vi "ConvertTextBasedCodeToLabVIEW_CreateOverviewHtmlFile.vi"(5 "InterfacesThatWillUseInheritance":string[](array[string]), 7 "MissingClasses":string[](array[string]), 8 "error in (no error)":errorcluster, 10 "Classes":T1[](array[typedef])=[{"ClassName"="Global", "AccessScope"=enum."public", "Modifiers"=[enum."static", enum."const"], "ClassDocumentation"="", "Methods"=[{"ReturnType"={"Name"="", "DataType"=enum."UINT8", "ArrayDim"=0, "CtrlPath"=path "", "DataTypeString"="", "AccessScope"=enum."public", "InitialData"=variant}, "MethodName"="", "AccessScope"=enum."public", "Modifiers"=[], "MethodDocumentation"="", "MethodContent"="", "MethodArguments"=[], "GetProperty"={"Active"=FALSE, "AccessScope"=enum."public", "Code"=""}, "SetProperty"={"Active"=FALSE, "AccessScope"=enum."public", "Code"=""}}], "ParentClasses"=[{"ClassName"="HttpApplication", "ClassType"=enum."Undefined"}], "ClassType"=enum."Class", "Owner"="", "OwnerType"=enum."NoOwner", "Generics"=["X", "Y"], "Attributes"=[{"Name"="Name", "DataType"=enum."STRING", "ArrayDim"=0, "CtrlPath"=path "", "DataTypeString"="", "AccessScope"=enum."public", "InitialData"=variant}, {"Name"="Points", "DataType"=enum."Other", "ArrayDim"=1, "CtrlPath"=path "", "DataTypeString"="", "AccessScope"=enum."protected", "InitialData"=variant}], "Enums"=[{"Name"="Alignment", "AccessScope"=enum."public", "Modifiers"=[], "Items"=["Top", "Left"], "Documentation"="This is doc"}], "Structs"=[{"Name"="MyStruct", "AccessScope"=enum."public", "Modifiers"=[enum."static"], "Items"=[{"Name"="A", "DataType"=enum."UINT8", "ArrayDim"=0, "CtrlPath"=path "", "DataTypeString"="", "AccessScope"=enum."public", "InitialData"=variant}, {"Name"="B", "DataType"=enum."INT32", "ArrayDim"=2, "CtrlPath"=path "", "DataTypeString"="", "AccessScope"=enum."public", "InitialData"=variant}], "Documentation"="Doc of My Strcutc\nBlah Blah YUmmi"}]}, {"ClassName"="ApplicationUser", "AccessScope"=enum."public", "Modifiers"=[], "ClassDocumentation"="You can add User data for the user by adding more properties to your User class, please visit http://    public", "Methods"=[{"ReturnType"={"Name"="", "DataType"=enum."UINT8", "ArrayDim"=0, "CtrlPath"=path "", "DataTypeString"="", "AccessScope"=enum."public", "InitialData"=variant}, "MethodName"="", "AccessScope"=enum."public", "Modifiers"=[], "MethodDocumentation"="", "MethodContent"="", "MethodArguments"=[], "GetProperty"={"Active"=FALSE, "AccessScope"=enum."public", "Code"=""}, "SetProperty"={"Active"=FALSE, "AccessScope"=enum."public", "Code"=""}}, {"ReturnType"={"Name"="", "DataType"=enum."UINT8", "ArrayDim"=0, "CtrlPath"=path "", "DataTypeString"="", "AccessScope"=enum."public", "InitialData"=variant}, "MethodName"="", "AccessScope"=enum."public", "Modifiers"=[], "MethodDocumentation"="", "MethodContent"="", "MethodArguments"=[], "GetProperty"={"Active"=FALSE, "AccessScope"=enum."public", "Code"=""}, "SetProperty"={"Active"=FALSE, "AccessScope"=enum."public", "Code"=""}}], "ParentClasses"=[{"ClassName"="IdentityUser", "ClassType"=enum."Undefined"}], "ClassType"=enum."Class", "Owner"="", "OwnerType"=enum."NoOwner", "Generics"=[], "Attributes"=[], "Enums"=[], "Structs"=[]}, {"ClassName"="ApplicationDbContext", "AccessScope"=enum."public", "Modifiers"=[], "ClassDocumentation"="", "Methods"=[{"ReturnType"={"Name"="", "DataType"=enum."UINT8", "ArrayDim"=0, "CtrlPath"=path "", "DataTypeString"="", "AccessScope"=enum."public", "InitialData"=variant}, "MethodName"="", "AccessScope"=enum."public", "Modifiers"=[], "MethodDocumentation"="", "MethodContent"="", "MethodArguments"=[], "GetProperty"={"Active"=FALSE, "AccessScope"=enum."public", "Code"=""}, "SetProperty"={"Active"=FALSE, "AccessScope"=enum."public", "Code"=""}}, {"ReturnType"={"Name"="", "DataType"=enum."UINT8", "ArrayDim"=0, "CtrlPath"=path "", "DataTypeString"="", "AccessScope"=enum."public", "InitialData"=variant}, "MethodName"="", "AccessScope"=enum."public", "Modifiers"=[], "MethodDocumentation"="", "MethodContent"="", "MethodArguments"=[], "GetProperty"={"Active"=FALSE, "AccessScope"=enum."public", "Code"=""}, "SetProperty"={"Active"=FALSE, "AccessScope"=enum."public", "Code"=""}}], "ParentClasses"=[{"ClassName"="IdentityDbContext", "ClassType"=enum."Undefined"}], "ClassType"=enum."Class", "Owner"="", "OwnerType"=enum."NoOwner", "Generics"=["ApplicationUser"], "Attributes"=[], "Enums"=[], "Structs"=[]}, {"ClassName"="IdentityHelper", "AccessScope"=enum."public", "Modifiers"=[enum."static"], "ClassDocumentation"="", "Methods"=[{"ReturnType"={"Name"="", "DataType"=enum."UINT8", "ArrayDim"=0, "CtrlPath"=path "", "DataTypeString"="", "AccessScope"=enum."public", "InitialData"=variant}, "MethodName"="", "AccessScope"=enum."public", "Modifiers"=[], "MethodDocumentation"="", "MethodContent"="", "MethodArguments"=[], "GetProperty"={"Active"=FALSE, "AccessScope"=enum."public", "Code"=""}, "SetProperty"={"Active"=FALSE, "AccessScope"=enum."public", "Code"=""}}, {"ReturnType"={"Name"="", "DataType"=enum."UINT8", "ArrayDim"=0, "CtrlPath"=path "", "DataTypeString"="", "AccessScope"=enum."public", "InitialData"=variant}, "MethodName"="", "AccessScope"=enum."public", "Modifiers"=[], "MethodDocumentation"="", "MethodContent"="", "MethodArguments"=[], "GetProperty"={"Active"=FALSE, "AccessScope"=enum."public", "Code"=""}, "SetProperty"={"Active"=FALSE, "AccessScope"=enum."public", "Code"=""}}, {"ReturnType"={"Name"="", "DataType"=enum."UINT8", "ArrayDim"=0, "CtrlPath"=path "", "DataTypeString"="", "AccessScope"=enum."public", "InitialData"=variant}, "MethodName"="", "AccessScope"=enum."public", "Modifiers"=[], "MethodDocumentation"="", "MethodContent"="", "MethodArguments"=[], "GetProperty"={"Active"=FALSE, "AccessScope"=enum."public", "Code"=""}, "SetProperty"={"Active"=FALSE, "AccessScope"=enum."public", "Code"=""}}, {"ReturnType"={"Name"="", "DataType"=enum."UINT8", "ArrayDim"=0, "CtrlPath"=path "", "DataTypeString"="", "AccessScope"=enum."public", "InitialData"=variant}, "MethodName"="", "AccessScope"=enum."public", "Modifiers"=[], "MethodDocumentation"="", "MethodContent"="", "MethodArguments"=[], "GetProperty"={"Active"=FALSE, "AccessScope"=enum."public", "Code"=""}, "SetProperty"={"Active"=FALSE, "AccessScope"=enum."public", "Code"=""}}, {"ReturnType"={"Name"="", "DataType"=enum."UINT8", "ArrayDim"=0, "CtrlPath"=path "", "DataTypeString"="", "AccessScope"=enum."public", "InitialData"=variant}, "MethodName"="", "AccessScope"=enum."public", "Modifiers"=[], "MethodDocumentation"="", "MethodContent"="", "MethodArguments"=[], "GetProperty"={"Active"=FALSE, "AccessScope"=enum."public", "Code"=""}, "SetProperty"={"Active"=FALSE, "AccessScope"=enum."public", "Code"=""}}, {"ReturnType"={"Name"="", "DataType"=enum."UINT8", "ArrayDim"=0, "CtrlPath"=path "", "DataTypeString"="", "AccessScope"=enum."public", "InitialData"=variant}, "MethodName"="", "AccessScope"=enum."public", "Modifiers"=[], "MethodDocumentation"="", "MethodContent"="", "MethodArguments"=[], "GetProperty"={"Active"=FALSE, "AccessScope"=enum."public", "Code"=""}, "SetProperty"={"Active"=FALSE, "AccessScope"=enum."public", "Code"=""}}, {"ReturnType"={"Name"="", "DataType"=enum."UINT8", "ArrayDim"=0, "CtrlPath"=path "", "DataTypeString"="", "AccessScope"=enum."public", "InitialData"=variant}, "MethodName"="", "AccessScope"=enum."public", "Modifiers"=[], "MethodDocumentation"="", "MethodContent"="", "MethodArguments"=[], "GetProperty"={"Active"=FALSE, "AccessScope"=enum."public", "Code"=""}, "SetProperty"={"Active"=FALSE, "AccessScope"=enum."public", "Code"=""}}, {"ReturnType"={"Name"="", "DataType"=enum."UINT8", "ArrayDim"=0, "CtrlPath"=path "", "DataTypeString"="", "AccessScope"=enum."public", "InitialData"=variant}, "MethodName"="", "AccessScope"=enum."public", "Modifiers"=[], "MethodDocumentation"="", "MethodContent"="", "MethodArguments"=[], "GetProperty"={"Active"=FALSE, "AccessScope"=enum."public", "Code"=""}, "SetProperty"={"Active"=FALSE, "AccessScope"=enum."public", "Code"=""}}], "ParentClasses"=[], "ClassType"=enum."Class", "Owner"="", "OwnerType"=enum."NoOwner", "Generics"=[], "Attributes"=[{"Name"="XsrfKey", "DataType"=enum."STRING", "ArrayDim"=0, "CtrlPath"=path "", "DataTypeString"="string", "AccessScope"=enum."public", "InitialData"=variant(string "\"XsrfId\"")}, {"Name"="ProviderNameKey", "DataType"=enum."STRING", "ArrayDim"=0, "CtrlPath"=path "", "DataTypeString"="string", "AccessScope"=enum."public", "InitialData"=variant(string "\"providerName\"")}, {"Name"="CodeKey", "DataType"=enum."STRING", "ArrayDim"=0, "CtrlPath"=path "", "DataTypeString"="string", "AccessScope"=enum."public", "InitialData"=variant(string "\"code\"")}, {"Name"="UserIdKey", "DataType"=enum."STRING", "ArrayDim"=0, "CtrlPath"=path "", "DataTypeString"="string", "AccessScope"=enum."public", "InitialData"=variant(string "\"userId\"")}], "Enums"=[], "Structs"=[]}, {"ClassName"="Register", "AccessScope"=enum."public", "Modifiers"=[enum."partial"], "ClassDocumentation"="", "Methods"=[{"ReturnType"={"Name"="", "DataType"=enum."UINT8", "ArrayDim"=0, "CtrlPath"=path "", "DataTypeString"="", "AccessScope"=enum."public", "InitialData"=variant}, "MethodName"="", "AccessScope"=enum."public", "Modifiers"=[], "MethodDocumentation"="", "MethodContent"="", "MethodArguments"=[], "GetProperty"={"Active"=FALSE, "AccessScope"=enum."public", "Code"=""}, "SetProperty"={"Active"=FALSE, "AccessScope"=enum."public", "Code"=""}}, {"ReturnType"={"Name"="", "DataType"=enum."UINT8", "ArrayDim"=0, "CtrlPath"=path "", "DataTypeString"="", "AccessScope"=enum."public", "InitialData"=variant}, "MethodName"="", "AccessScope"=enum."public", "Modifiers"=[], "MethodDocumentation"="", "MethodContent"="", "MethodArguments"=[], "GetProperty"={"Active"=FALSE, "AccessScope"=enum."public", "Code"=""}, "SetProperty"={"Active"=FALSE, "AccessScope"=enum."public", "Code"=""}}], "ParentClasses"=[{"ClassName"="Page", "ClassType"=enum."Undefined"}], "ClassType"=enum."Class", "Owner"="", "OwnerType"=enum."NoOwner", "Generics"=[], "Attributes"=[], "Enums"=[], "Structs"=[]}, {"ClassName"="RoleActions", "AccessScope"=enum."internal", "Modifiers"=[], "ClassDocumentation"="", "Methods"=[{"ReturnType"={"Name"="", "DataType"=enum."UINT8", "ArrayDim"=0, "CtrlPath"=path "", "DataTypeString"="", "AccessScope"=enum."public", "InitialData"=variant}, "MethodName"="", "AccessScope"=enum."public", "Modifiers"=[], "MethodDocumentation"="", "MethodContent"="", "MethodArguments"=[], "GetProperty"={"Active"=FALSE, "AccessScope"=enum."public", "Code"=""}, "SetProperty"={"Active"=FALSE, "AccessScope"=enum."public", "Code"=""}}], "ParentClasses"=[], "ClassType"=enum."Class", "Owner"="", "OwnerType"=enum."NoOwner", "Generics"=[], "Attributes"=[], "Enums"=[], "Structs"=[]}, {"ClassName"="SugiyamaLayout", "AccessScope"=enum."public", "Modifiers"=[], "ClassDocumentation"="Arranges the nodes with the Sugiyama Layout Algorithm.<br>\n\n<a href=\"http://plg.uwaterloo.ca/~itbowman/CS746G/Notes/Sugiyama1981_MVU/\">\nLink to the algorithm</a>\n\n<br>\n<br>\n@author Sven Luzar<br>\nmodified by Gaudenz Alder\n@version 1.0 init", "Methods"=[{"ReturnType"={"Name"="", "DataType"=enum."UINT8", "ArrayDim"=0, "CtrlPath"=path "", "DataTypeString"="", "AccessScope"=enum."public", "InitialData"=variant}, "MethodName"="", "AccessScope"=enum."public", "Modifiers"=[], "MethodDocumentation"="", "MethodContent"="", "MethodArguments"=[], "GetProperty"={"Active"=FALSE, "AccessScope"=enum."public", "Code"=""}, "SetProperty"={"Active"=FALSE, "AccessScope"=enum."public", "Code"=""}}, {"ReturnType"={"Name"="", "DataType"=enum."UINT8", "ArrayDim"=0, "CtrlPath"=path "", "DataTypeString"="", "AccessScope"=enum."public", "InitialData"=variant}, "MethodName"="", "AccessScope"=enum."public", "Modifiers"=[], "MethodDocumentation"="", "MethodContent"="", "MethodArguments"=[], "GetProperty"={"Active"=FALSE, "AccessScope"=enum."public", "Code"=""}, "SetProperty"={"Active"=FALSE, "AccessScope"=enum."public", "Code"=""}}, {"ReturnType"={"Name"="", "DataType"=enum."UINT8", "ArrayDim"=0, "CtrlPath"=path "", "DataTypeString"="", "AccessScope"=enum."public", "InitialData"=variant}, "MethodName"="", "AccessScope"=enum."public", "Modifiers"=[], "MethodDocumentation"="", "MethodContent"="", "MethodArguments"=[], "GetProperty"={"Active"=FALSE, "AccessScope"=enum."public", "Code"=""}, "SetProperty"={"Active"=FALSE, "AccessScope"=enum."public", "Code"=""}}, {"ReturnType"={"Name"="", "DataType"=enum."UINT8", "ArrayDim"=0, "CtrlPath"=path "", "DataTypeString"="", "AccessScope"=enum."public", "InitialData"=variant}, "MethodName"="", "AccessScope"=enum."public", "Modifiers"=[], "MethodDocumentation"="", "MethodContent"="", "MethodArguments"=[], "GetProperty"={"Active"=FALSE, "AccessScope"=enum."public", "Code"=""}, "SetProperty"={"Active"=FALSE, "AccessScope"=enum."public", "Code"=""}}, {"ReturnType"={"Name"="", "DataType"=enum."UINT8", "ArrayDim"=0, "CtrlPath"=path "", "DataTypeString"="", "AccessScope"=enum."public", "InitialData"=variant}, "MethodName"="", "AccessScope"=enum."public", "Modifiers"=[], "MethodDocumentation"="", "MethodContent"="", "MethodArguments"=[], "GetProperty"={"Active"=FALSE, "AccessScope"=enum."public", "Code"=""}, "SetProperty"={"Active"=FALSE, "AccessScope"=enum."public", "Code"=""}}, {"ReturnType"={"Name"="", "DataType"=enum."UINT8", "ArrayDim"=0, "CtrlPath"=path "", "DataTypeString"="", "AccessScope"=enum."public", "InitialData"=variant}, "MethodName"="", "AccessScope"=enum."public", "Modifiers"=[], "MethodDocumentation"="", "MethodContent"="", "MethodArguments"=[], "GetProperty"={"Active"=FALSE, "AccessScope"=enum."public", "Code"=""}, "SetProperty"={"Active"=FALSE, "AccessScope"=enum."public", "Code"=""}}, {"ReturnType"={"Name"="", "DataType"=enum."UINT8", "ArrayDim"=0, "CtrlPath"=path "", "DataTypeString"="", "AccessScope"=enum."public", "InitialData"=variant}, "MethodName"="", "AccessScope"=enum."public", "Modifiers"=[], "MethodDocumentation"="", "MethodContent"="", "MethodArguments"=[], "GetProperty"={"Active"=FALSE, "AccessScope"=enum."public", "Code"=""}, "SetProperty"={"Active"=FALSE, "AccessScope"=enum."public", "Code"=""}}, {"ReturnType"={"Name"="", "DataType"=enum."UINT8", "ArrayDim"=0, "CtrlPath"=path "", "DataTypeString"="", "AccessScope"=enum."public", "InitialData"=variant}, "MethodName"="", "AccessScope"=enum."public", "Modifiers"=[], "MethodDocumentation"="", "MethodContent"="", "MethodArguments"=[], "GetProperty"={"Active"=FALSE, "AccessScope"=enum."public", "Code"=""}, "SetProperty"={"Active"=FALSE, "AccessScope"=enum."public", "Code"=""}}, {"ReturnType"={"Name"="", "DataType"=enum."UINT8", "ArrayDim"=0, "CtrlPath"=path "", "DataTypeString"="", "AccessScope"=enum."public", "InitialData"=variant}, "MethodName"="", "AccessScope"=enum."public", "Modifiers"=[], "MethodDocumentation"="", "MethodContent"="", "MethodArguments"=[], "GetProperty"={"Active"=FALSE, "AccessScope"=enum."public", "Code"=""}, "SetProperty"={"Active"=FALSE, "AccessScope"=enum."public", "Code"=""}}, {"ReturnType"={"Name"="", "DataType"=enum."UINT8", "ArrayDim"=0, "CtrlPath"=path "", "DataTypeString"="", "AccessScope"=enum."public", "InitialData"=variant}, "MethodName"="", "AccessScope"=enum."public", "Modifiers"=[], "MethodDocumentation"="", "MethodContent"="", "MethodArguments"=[], "GetProperty"={"Active"=FALSE, "AccessScope"=enum."public", "Code"=""}, "SetProperty"={"Active"=FALSE, "AccessScope"=enum."public", "Code"=""}}, {"ReturnType"={"Name"="", "DataType"=enum."UINT8", "ArrayDim"=0, "CtrlPath"=path "", "DataTypeString"="", "AccessScope"=enum."public", "InitialData"=variant}, "MethodName"="", "AccessScope"=enum."public", "Modifiers"=[], "MethodDocumentation"="", "MethodContent"="", "MethodArguments"=[], "GetProperty"={"Active"=FALSE, "AccessScope"=enum."public", "Code"=""}, "SetProperty"={"Active"=FALSE, "AccessScope"=enum."public", "Code"=""}}, {"ReturnType"={"Name"="", "DataType"=enum."UINT8", "ArrayDim"=0, "CtrlPath"=path "", "DataTypeString"="", "AccessScope"=enum."public", "InitialData"=variant}, "MethodName"="", "AccessScope"=enum."public", "Modifiers"=[], "MethodDocumentation"="", "MethodContent"="", "MethodArguments"=[], "GetProperty"={"Active"=FALSE, "AccessScope"=enum."public", "Code"=""}, "SetProperty"={"Active"=FALSE, "AccessScope"=enum."public", "Code"=""}}, {"ReturnType"={"Name"="", "DataType"=enum."UINT8", "ArrayDim"=0, "CtrlPath"=path "", "DataTypeString"="", "AccessScope"=enum."public", "InitialData"=variant}, "MethodName"="", "AccessScope"=enum."public", "Modifiers"=[], "MethodDocumentation"="", "MethodContent"="", "MethodArguments"=[], "GetProperty"={"Active"=FALSE, "AccessScope"=enum."public", "Code"=""}, "SetProperty"={"Active"=FALSE, "AccessScope"=enum."public", "Code"=""}}, {"ReturnType"={"Name"="", "DataType"=enum."UINT8", "ArrayDim"=0, "CtrlPath"=path "", "DataTypeString"="", "AccessScope"=enum."public", "InitialData"=variant}, "MethodName"="", "AccessScope"=enum."public", "Modifiers"=[], "MethodDocumentation"="", "MethodContent"="", "MethodArguments"=[], "GetProperty"={"Active"=FALSE, "AccessScope"=enum."public", "Code"=""}, "SetProperty"={"Active"=FALSE, "AccessScope"=enum."public", "Code"=""}}, {"ReturnType"={"Name"="", "DataType"=enum."UINT8", "ArrayDim"=0, "CtrlPath"=path "", "DataTypeString"="", "AccessScope"=enum."public", "InitialData"=variant}, "MethodName"="", "AccessScope"=enum."public", "Modifiers"=[], "MethodDocumentation"="", "MethodContent"="", "MethodArguments"=[], "GetProperty"={"Active"=FALSE, "AccessScope"=enum."public", "Code"=""}, "SetProperty"={"Active"=FALSE, "AccessScope"=enum."public", "Code"=""}}, {"ReturnType"={"Name"="", "DataType"=enum."UINT8", "ArrayDim"=0, "CtrlPath"=path "", "DataTypeString"="", "AccessScope"=enum."public", "InitialData"=variant}, "MethodName"="", "AccessScope"=enum."public", "Modifiers"=[], "MethodDocumentation"="", "MethodContent"="", "MethodArguments"=[], "GetProperty"={"Active"=FALSE, "AccessScope"=enum."public", "Code"=""}, "SetProperty"={"Active"=FALSE, "AccessScope"=enum."public", "Code"=""}}, {"ReturnType"={"Name"="", "DataType"=enum."UINT8", "ArrayDim"=0, "CtrlPath"=path "", "DataTypeString"="", "AccessScope"=enum."public", "InitialData"=variant}, "MethodName"="", "AccessScope"=enum."public", "Modifiers"=[], "MethodDocumentation"="", "MethodContent"="", "MethodArguments"=[], "GetProperty"={"Active"=FALSE, "AccessScope"=enum."public", "Code"=""}, "SetProperty"={"Active"=FALSE, "AccessScope"=enum."public", "Code"=""}}, {"ReturnType"={"Name"="", "DataType"=enum."UINT8", "ArrayDim"=0, "CtrlPath"=path "", "DataTypeString"="", "AccessScope"=enum."public", "InitialData"=variant}, "MethodName"="", "AccessScope"=enum."public", "Modifiers"=[], "MethodDocumentation"="", "MethodContent"="", "MethodArguments"=[], "GetProperty"={"Active"=FALSE, "AccessScope"=enum."public", "Code"=""}, "SetProperty"={"Active"=FALSE, "AccessScope"=enum."public", "Code"=""}}, {"ReturnType"={"Name"="", "DataType"=enum."UINT8", "ArrayDim"=0, "CtrlPath"=path "", "DataTypeString"="", "AccessScope"=enum."public", "InitialData"=variant}, "MethodName"="", "AccessScope"=enum."public", "Modifiers"=[], "MethodDocumentation"="", "MethodContent"="", "MethodArguments"=[], "GetProperty"={"Active"=FALSE, "AccessScope"=enum."public", "Code"=""}, "SetProperty"={"Active"=FALSE, "AccessScope"=enum."public", "Code"=""}}, {"ReturnType"={"Name"="", "DataType"=enum."UINT8", "ArrayDim"=0, "CtrlPath"=path "", "DataTypeString"="", "AccessScope"=enum."public", "InitialData"=variant}, "MethodName"="", "AccessScope"=enum."public", "Modifiers"=[], "MethodDocumentation"="", "MethodContent"="", "MethodArguments"=[], "GetProperty"={"Active"=FALSE, "AccessScope"=enum."public", "Code"=""}, "SetProperty"={"Active"=FALSE, "AccessScope"=enum."public", "Code"=""}}, {"ReturnType"={"Name"="", "DataType"=enum."UINT8", "ArrayDim"=0, "CtrlPath"=path "", "DataTypeString"="", "AccessScope"=enum."public", "InitialData"=variant}, "MethodName"="", "AccessScope"=enum."public", "Modifiers"=[], "MethodDocumentation"="", "MethodContent"="", "MethodArguments"=[], "GetProperty"={"Active"=FALSE, "AccessScope"=enum."public", "Code"=""}, "SetProperty"={"Active"=FALSE, "AccessScope"=enum."public", "Code"=""}}, {"ReturnType"={"Name"="", "DataType"=enum."UINT8", "ArrayDim"=0, "CtrlPath"=path "", "DataTypeString"="", "AccessScope"=enum."public", "InitialData"=variant}, "MethodName"="", "AccessScope"=enum."public", "Modifiers"=[], "MethodDocumentation"="", "MethodContent"="", "MethodArguments"=[], "GetProperty"={"Active"=FALSE, "AccessScope"=enum."public", "Code"=""}, "SetProperty"={"Active"=FALSE, "AccessScope"=enum."public", "Code"=""}}], "ParentClasses"=[], "ClassType"=enum."Class", "Owner"="", "OwnerType"=enum."NoOwner", "Generics"=[], "Attributes"=[{"Name"="SUGIYAMA_VISITED", "DataType"=enum."STRING", "ArrayDim"=0, "CtrlPath"=path "", "DataTypeString"="String", "AccessScope"=enum."public", "InitialData"=variant(string "\"SugiyamaVisited\" /*#Frozen*/")}, {"Name"="SUGIYAMA_CELL_WRAPPER", "DataType"=enum."STRING", "ArrayDim"=0, "CtrlPath"=path "", "DataTypeString"="String", "AccessScope"=enum."public", "InitialData"=variant(string "\"SugiyamaCellWrapper\" /*#Frozen*/")}, {"Name"="gridAreaSize", "DataType"=enum."INT32", "ArrayDim"=0, "CtrlPath"=path "", "DataTypeString"="int", "AccessScope"=enum."protected", "InitialData"=variant(string "Integer.MIN_VALUE")}, {"Name"="movements", "DataType"=enum."Other", "ArrayDim"=0, "CtrlPath"=path "", "DataTypeString"="Vector", "AccessScope"=enum."private", "InitialData"=variant(string "null")}, {"Name"="movementsCurrentLoop", "DataType"=enum."INT32", "ArrayDim"=0, "CtrlPath"=path "", "DataTypeString"="int", "AccessScope"=enum."private", "InitialData"=variant(string "-1")}, {"Name"="movementsMax", "DataType"=enum."INT32", "ArrayDim"=0, "CtrlPath"=path "", "DataTypeString"="int", "AccessScope"=enum."private", "InitialData"=variant(string "Integer.MIN_VALUE")}, {"Name"="iteration", "DataType"=enum."INT32", "ArrayDim"=0, "CtrlPath"=path "", "DataTypeString"="int", "AccessScope"=enum."private", "InitialData"=variant(string "0")}, {"Name"="vertical", "DataType"=enum."BOOL", "ArrayDim"=0, "CtrlPath"=path "", "DataTypeString"="boolean", "AccessScope"=enum."protected", "InitialData"=variant(string "true")}, {"Name"="spacing", "DataType"=enum."Other", "ArrayDim"=0, "CtrlPath"=path "", "DataTypeString"="Point", "AccessScope"=enum."protected", "InitialData"=variant(string "new Point(250, 150)")}, {"Name"="wrappers", "DataType"=enum."Other", "ArrayDim"=0, "CtrlPath"=path "", "DataTypeString"="HashMap", "AccessScope"=enum."private", "InitialData"=variant(string "new HashMap()")}], "Enums"=[], "Structs"=[]}], 11 "appended path in":path=path "c:/Temp/ConvertTextToLV_Overview.html") -> (0 "error out":errorcluster, 3 "appended path out":path=path "C:/Users/mikael.holmstrom/AppData/Local/Temp/ConvertTextToLV_Overview.html")   [LabVIEW 2020]
uses:
  <resource>/Framework/Providers/Open_GDS/ClassProviders/Common/String/GDSString_ClassDescriptionType.ctl
  <resource>/Framework/Providers/Open_GDS/ClassProviders/Common/String/GDSString_AccessScopeModifierType.ctl
  <resource>/Framework/Providers/Open_GDS/ClassProviders/Common/String/GDSString_ModifierType.ctl
  <resource>/Framework/Providers/Open_GDS/ClassProviders/Common/String/GDSString_MethodDescriptionType.ctl
  <resource>/Framework/Providers/Open_GDS/ClassProviders/Common/CommonVIs/CommonVIs_AttributeType.ctl
  <resource>/Framework/Providers/Open_GDS/ClassProviders/Common/CommonVIs/CommonVIs_AttributeDataType.ctl
  <resource>/Framework/Providers/Open_GDS/ClassProviders/Common/CommonVIs/CommonVIs_PropertyType.ctl
  <resource>/Framework/Providers/Open_GDS/ClassProviders/Common/String/GDSString_ClassParentType.ctl
  <resource>/Framework/Providers/Open_GDS/ClassProviders/Common/String/GDSString_ClassType.ctl
  <resource>/Framework/Providers/Open_GDS/ClassProviders/Common/String/GDSString_ClassOwnerType.ctl
  <resource>/Framework/Providers/Open_GDS/ClassProviders/Common/CommonVIs/CommonVIs_EnumType.ctl
  <resource>/Framework/Providers/Open_GDS/ClassProviders/Common/CommonVIs/CommonVIs_StructType.ctl
  <vilib>/Platform/browser.llb/Open URL in Default Browser (path).vi
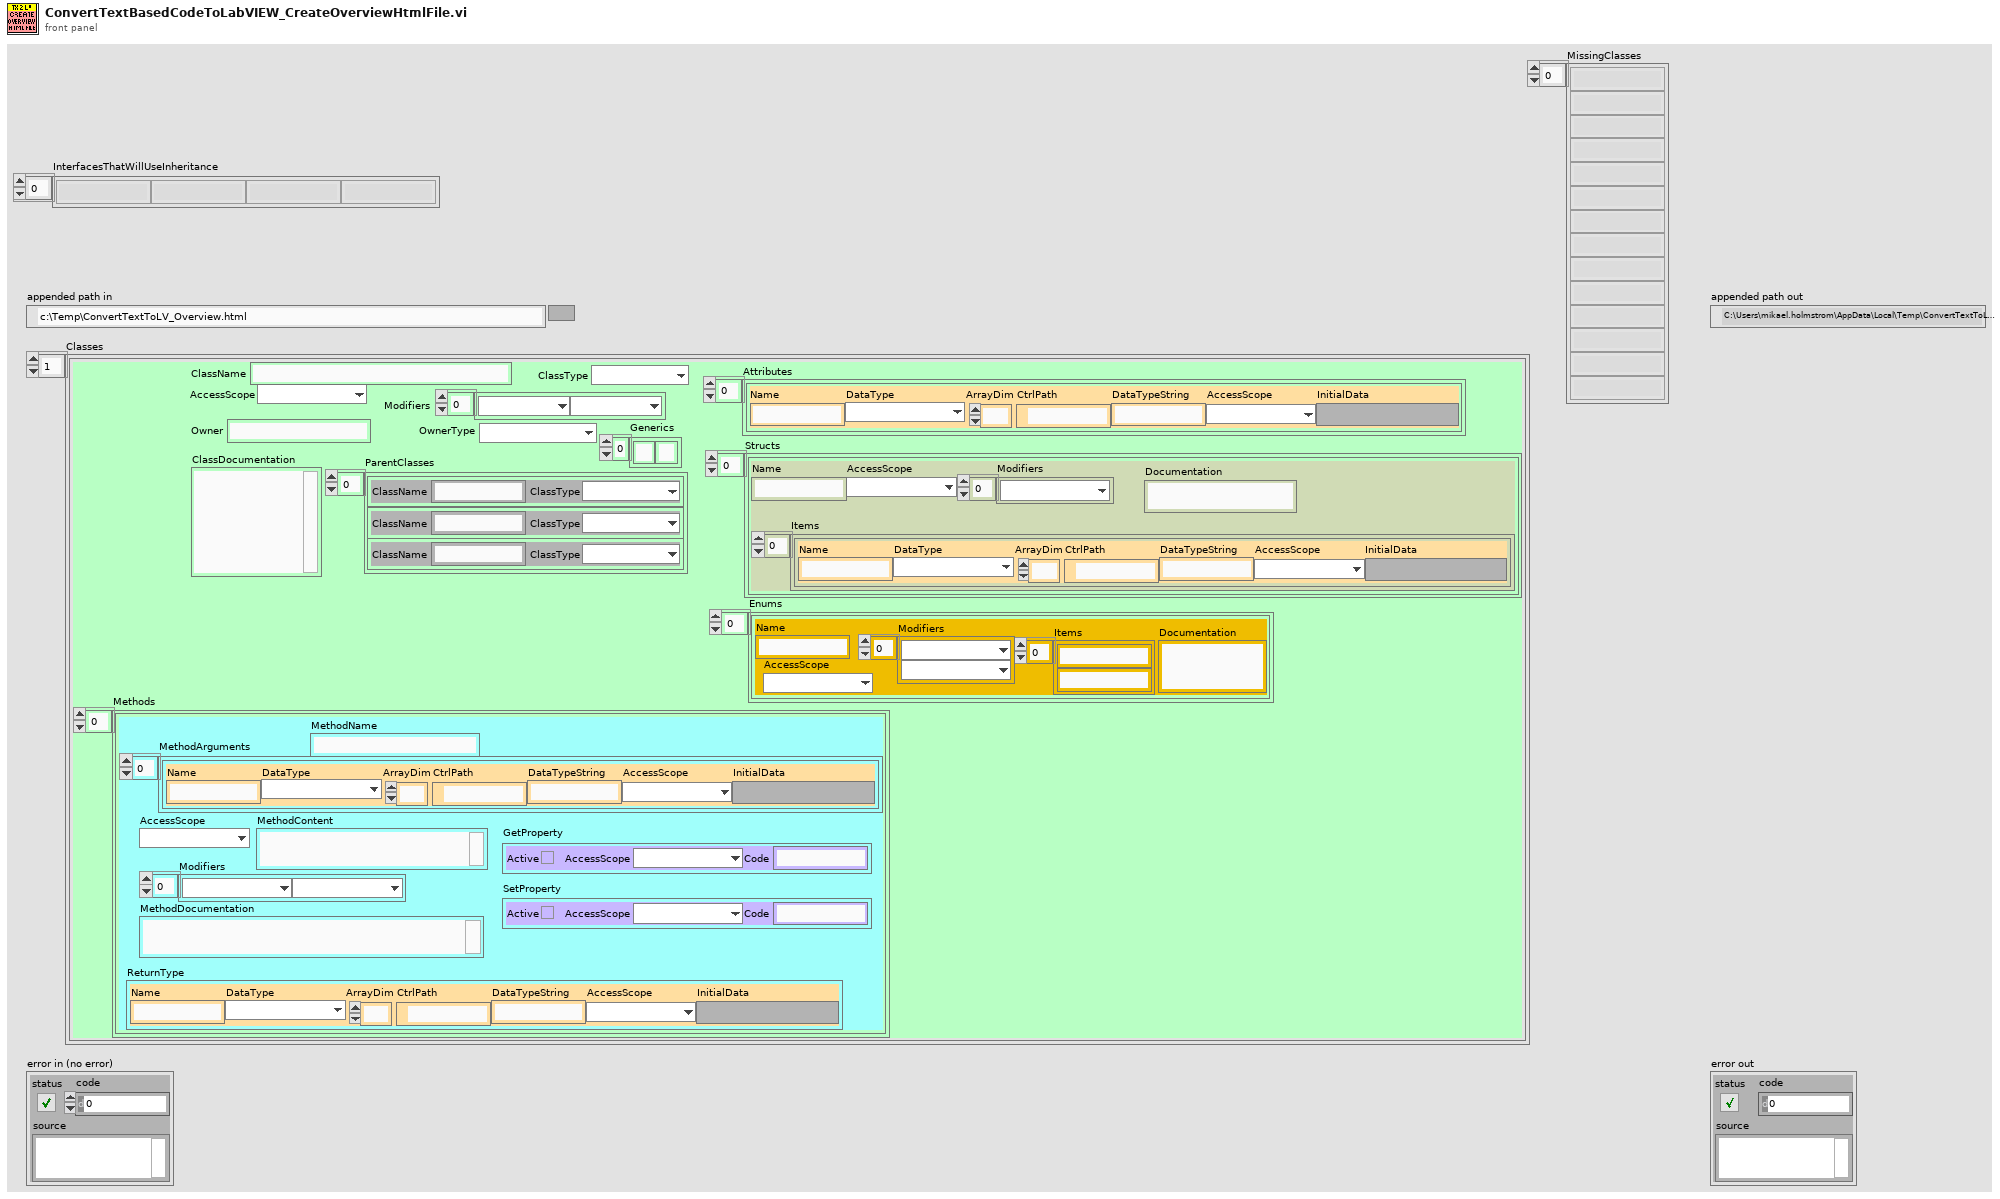
[diagram p1: front panel]
types:
  T1 = typedef "GDSString_ClassDescriptionType.ctl" = cluster{"ClassName":string, "AccessScope":T2, "Modifiers":T3[], "ClassDocumentation":string, "Methods":T4[], "ParentClasses":T8[], "ClassType":T9, "Owner":string, "OwnerType":T10, "Generics":string[], "Attributes":T5[], "Enums":T11[], "Structs":T12[]}
  T2 = typedef "GDSString_AccessScopeModifierType.ctl" = enum16{"public", "private", "protected", "internal"}
  T3 = typedef "GDSString_ModifierType.ctl" = enum16{"abstract", "static", "final", "synchronized", "strictfp", "async", "const", "event", "extern", "new", "native ", "override", "partial", "readonly", "sealed", "unsafe", "virtual", "volatile"}
  T4 = typedef "GDSString_MethodDescriptionType.ctl" = cluster{"ReturnType":T5, "MethodName":string, "AccessScope":T2, "Modifiers":T3[], "MethodDocumentation":string, "MethodContent":string, "MethodArguments":T5[], "GetProperty":T7, "SetProperty":T7}
  T5 = typedef "CommonVIs_AttributeType.ctl" = cluster{"Name":string, "DataType":T6, "ArrayDim":i32, "CtrlPath":path, "DataTypeString":string, "AccessScope":T2, "InitialData":variant}
  T6 = typedef "CommonVIs_AttributeDataType.ctl" = enum16{"UINT8", "INT8", "UINT16", "INT16", "UINT32", "INT32", "UINT64", "INT64", "SGL", "DBL", "EXT", "CSG", "CDB", "CXT", "TimeStamp", "STRING", "PATH", "BOOL", "ENUM", "RefNum", "VIRefNum", "LabVIEW Class", "Cluster", "Variant", "TypeDef", "Waveform", "LabVIEW Object", "Other", "void"}
  T7 = typedef "CommonVIs_PropertyType.ctl" = cluster{"Active":bool, "AccessScope":T2, "Code":string}
  T8 = typedef "GDSString_ClassParentType.ctl" = cluster{"ClassName":string, "ClassType":T9}
  T9 = typedef "GDSString_ClassType.ctl" = enum16{"Undefined", "Class", "Interface"}
  T10 = typedef "GDSString_ClassOwnerType.ctl" = enum16{"NoOwner", "Class", "Package/NameSpace"}
  T11 = typedef "CommonVIs_EnumType.ctl" = cluster{"Name":string, "AccessScope":T2, "Modifiers":T3[], "Items":string[], "Documentation":string}
  T12 = typedef "CommonVIs_StructType.ctl" = cluster{"Name":string, "AccessScope":T2, "Modifiers":T3[], "Items":T5[], "Documentation":string}
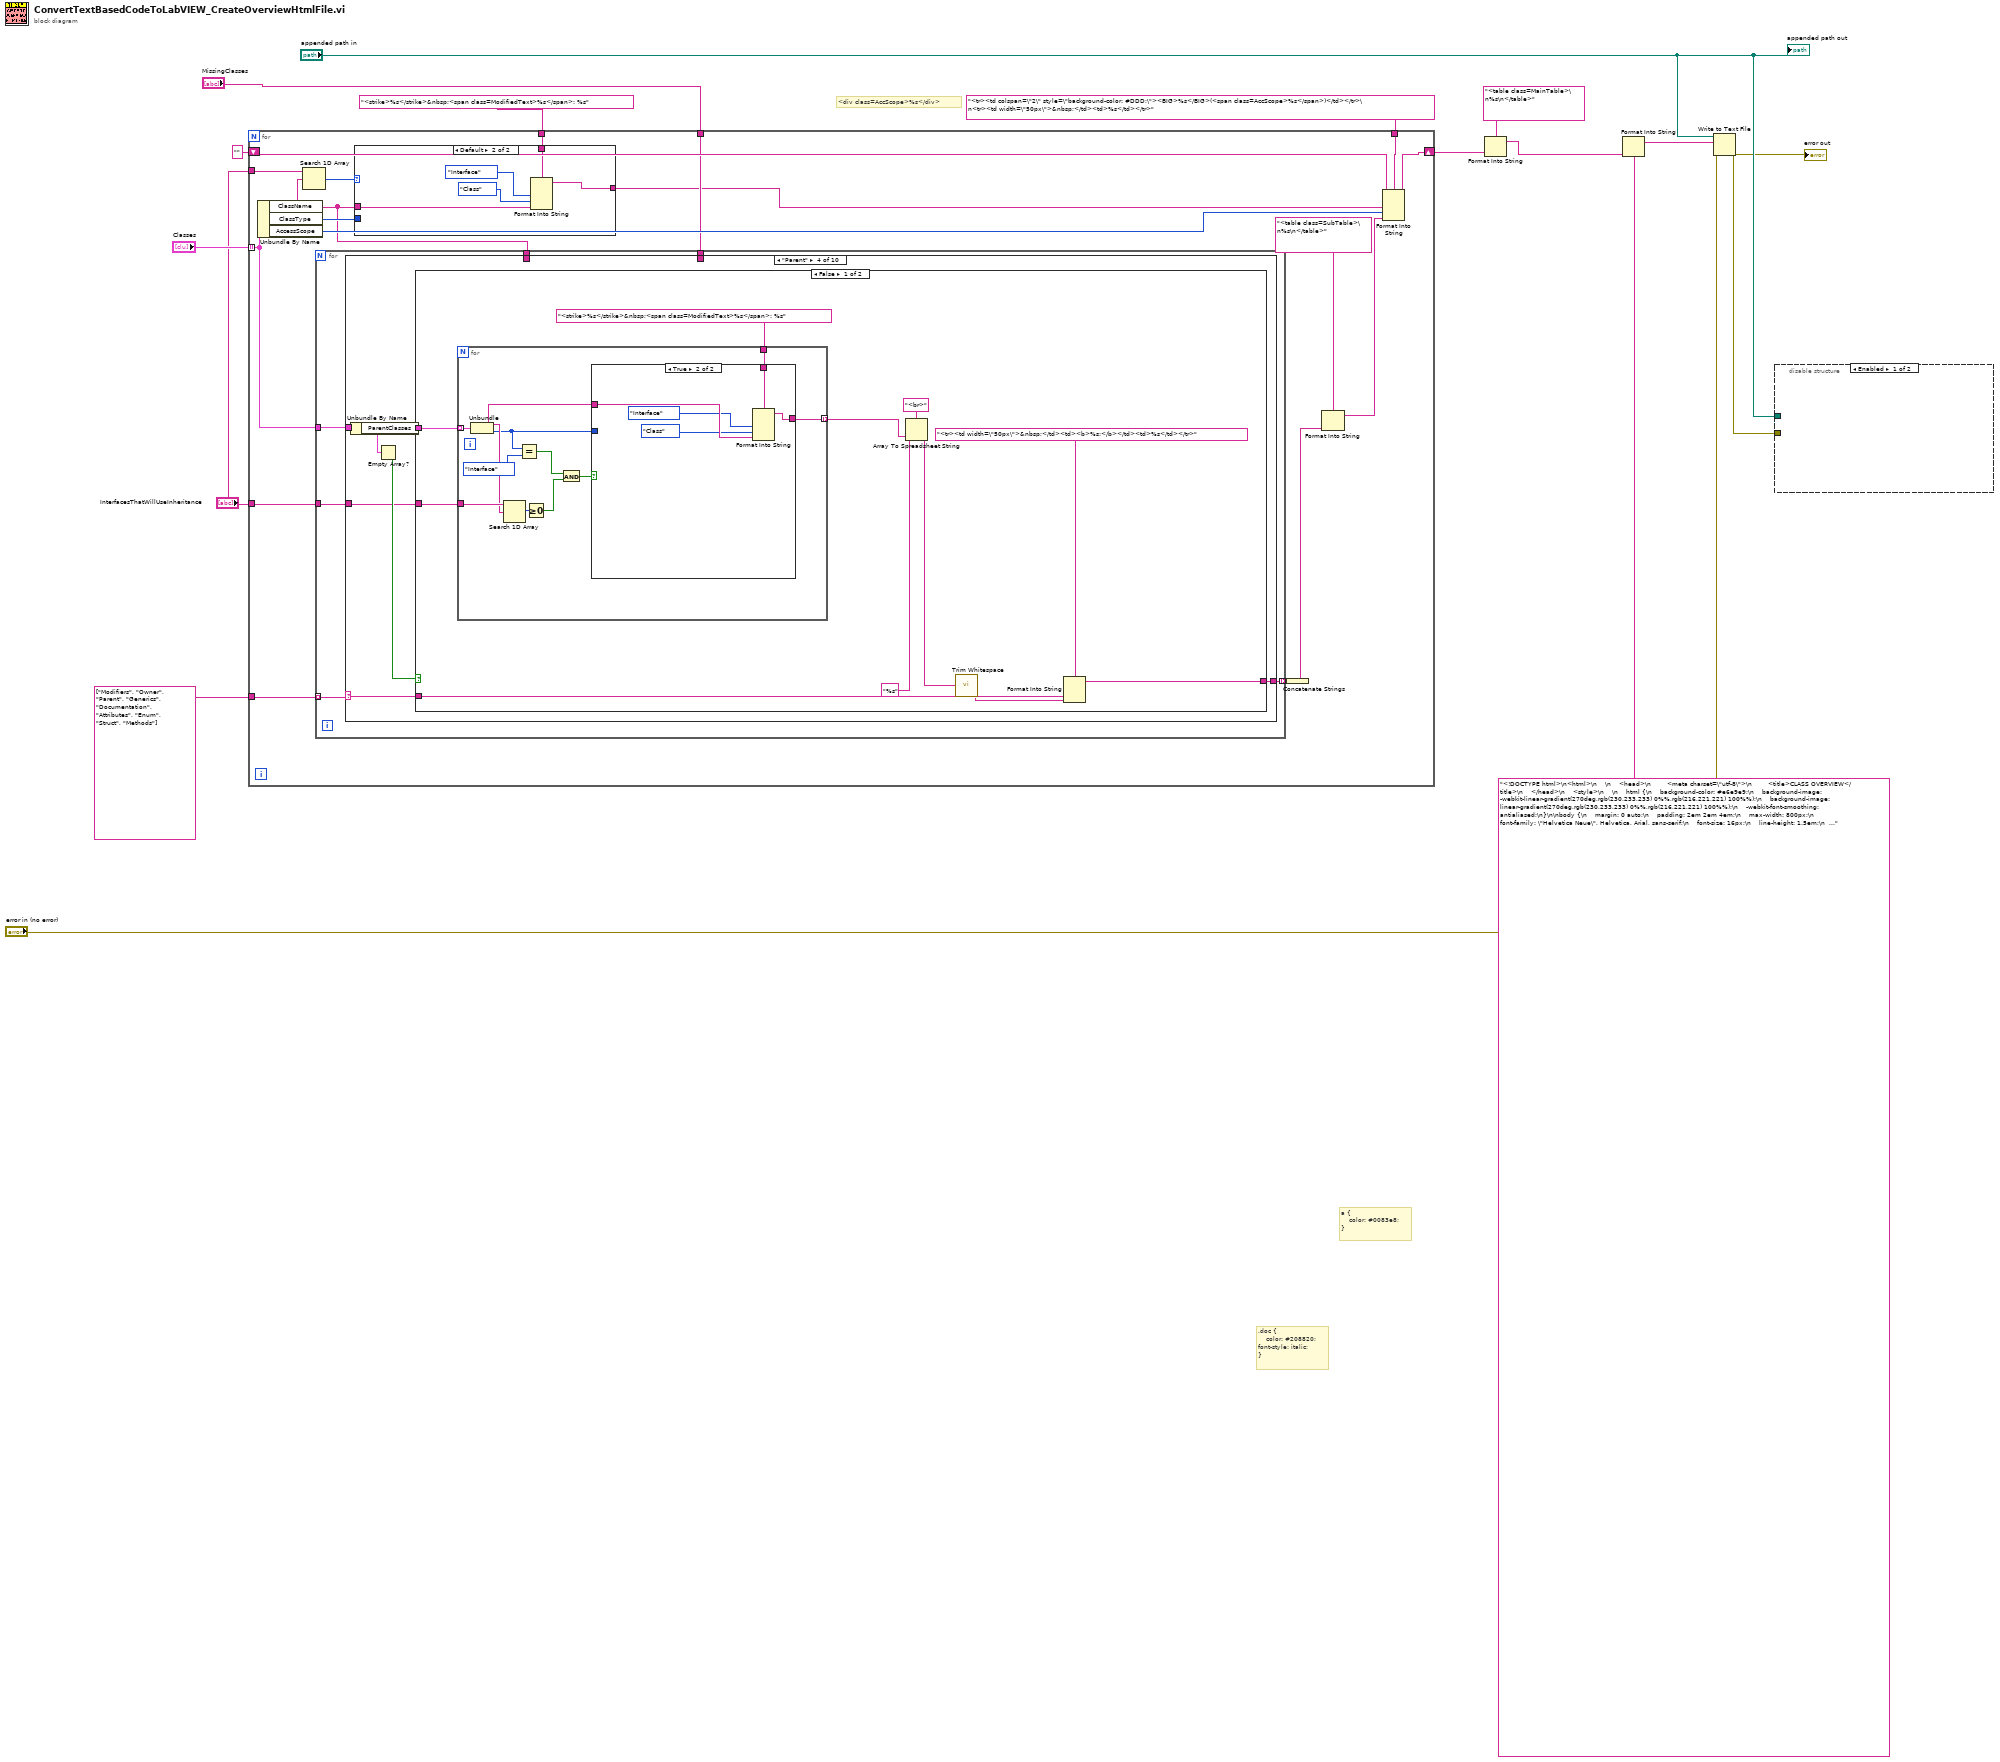
[diagram p0: block diagram]
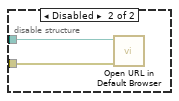
[diagram p2: hidden frame]
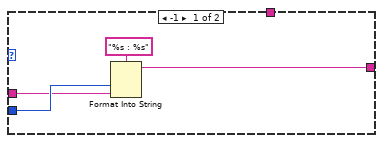
[diagram p3: hidden frame]
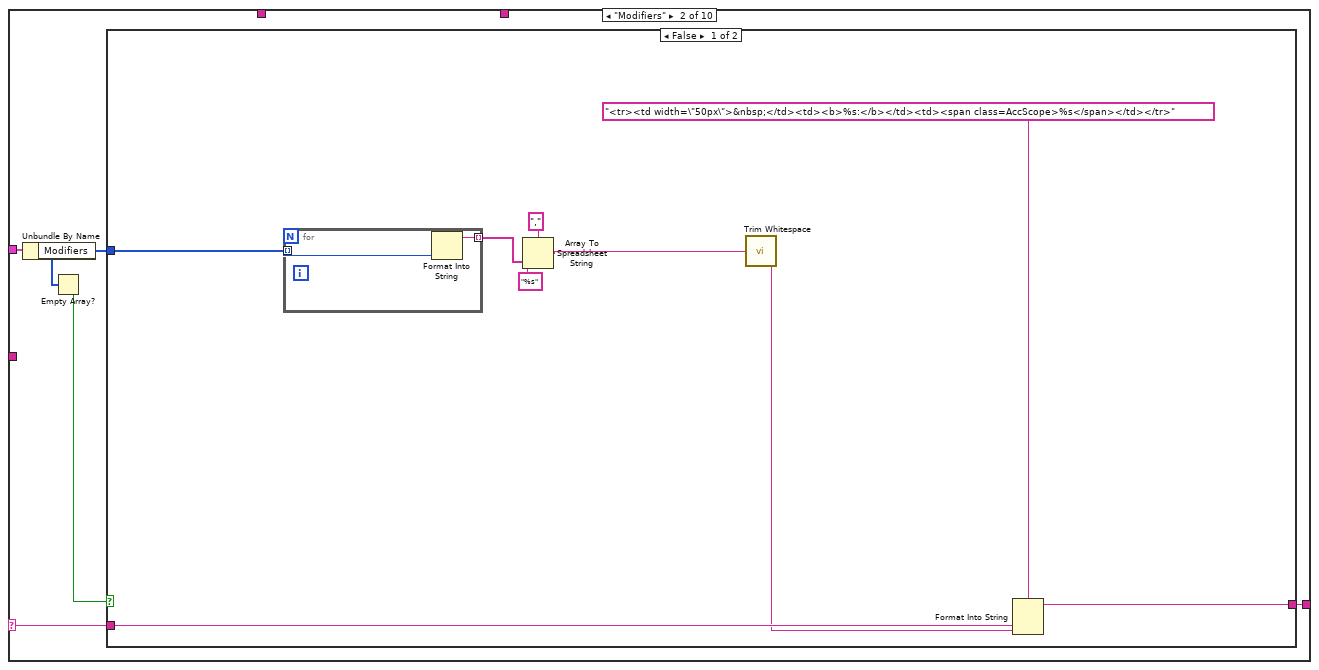
[diagram p5: hidden frame]
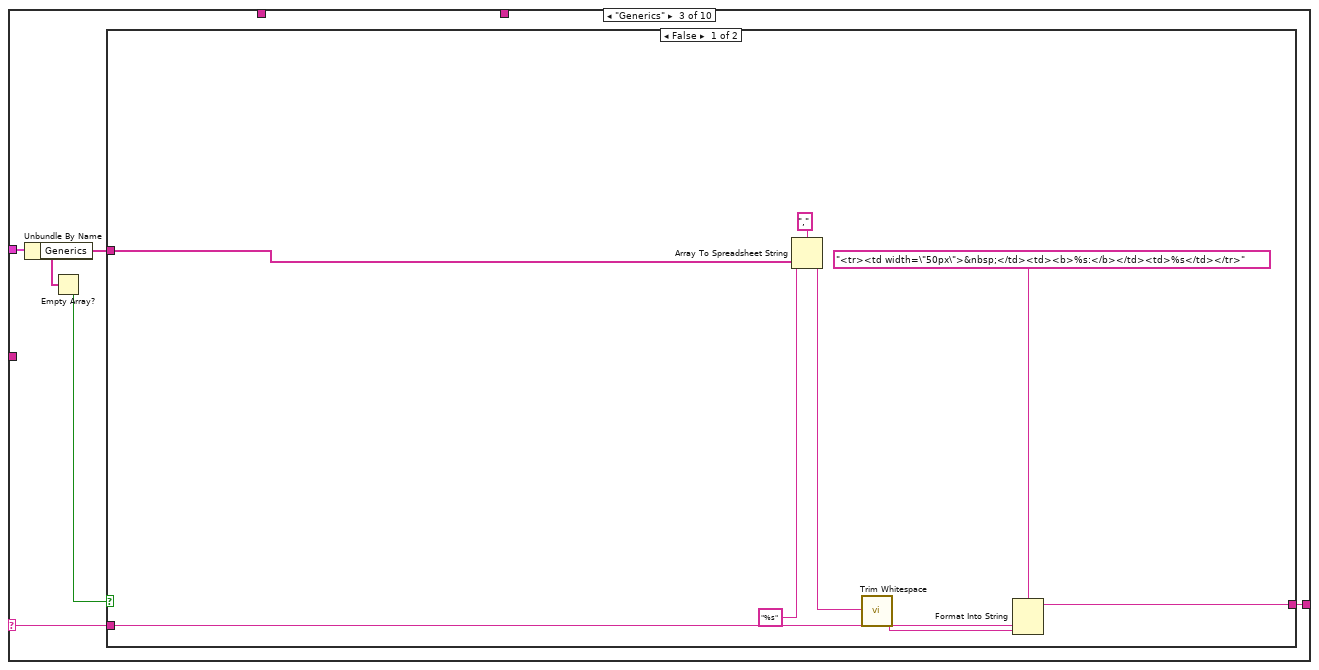
[diagram p7: hidden frame]
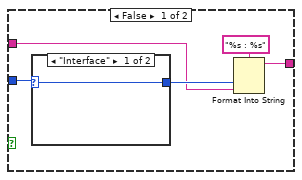
[diagram p9: hidden frame]
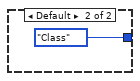
[diagram p10: hidden frame]
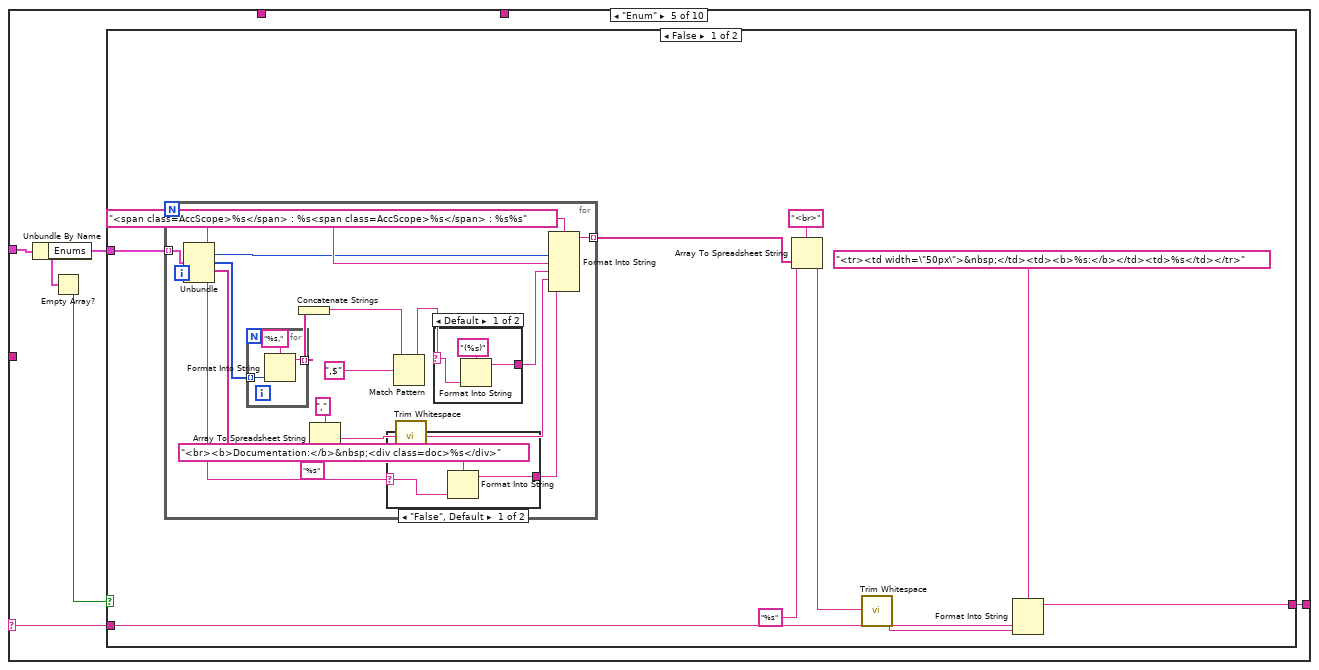
[diagram p12: hidden frame]
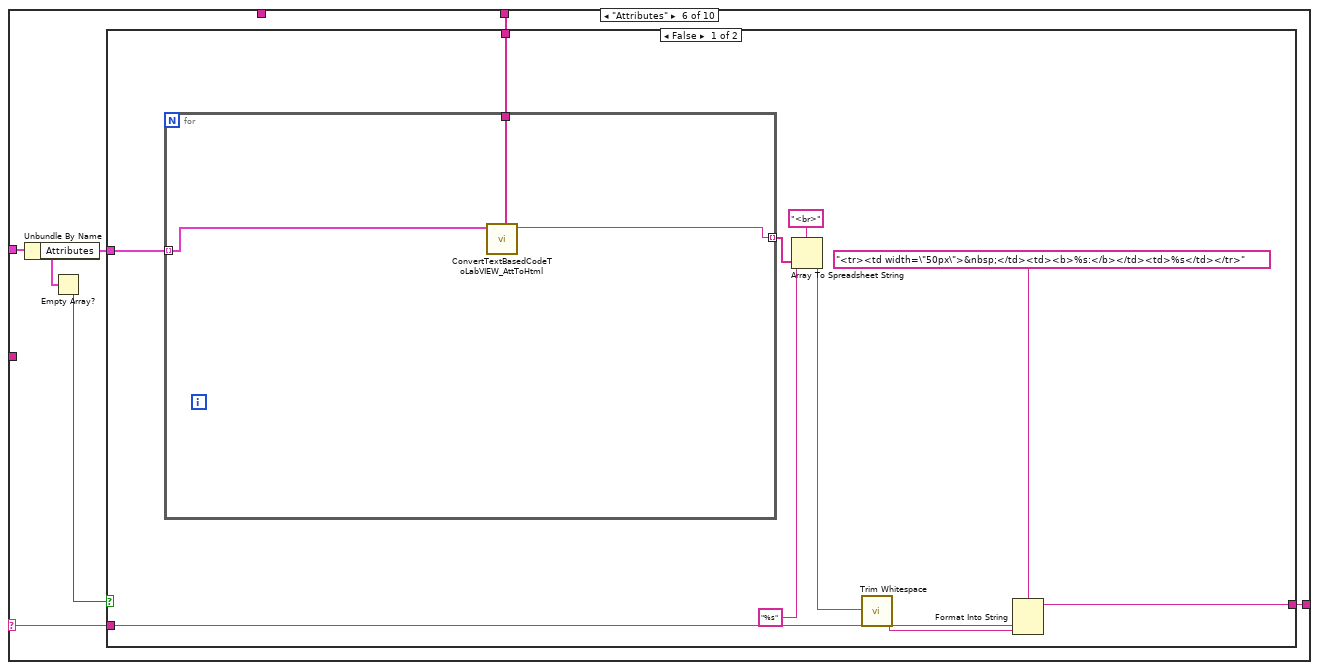
[diagram p16: hidden frame]
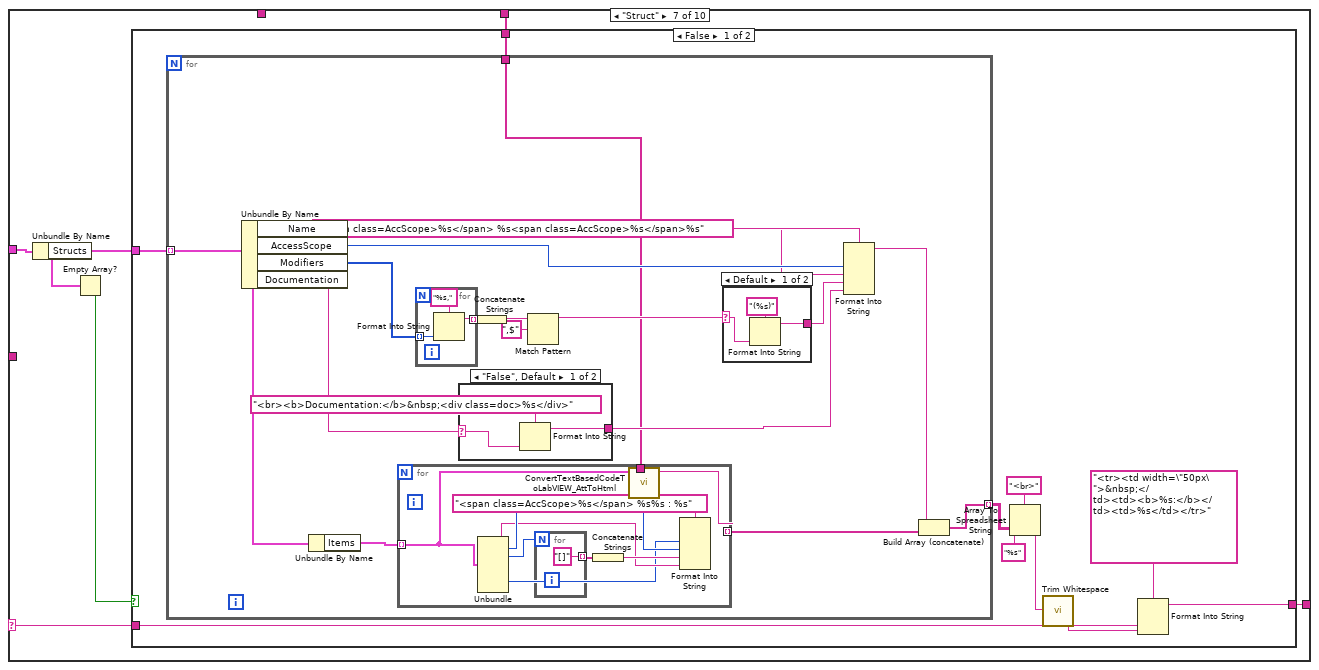
[diagram p18: hidden frame]
diagram:
  # ".doc {\n    color: #208820;\nfont-style: italic;\n}"
  # "<div class=AccScope>%s</div>"
  # "a {\n    color: #0083e8;\n}"
  n1 = for {
    tunnel: "Classes" -> [w27] mode=indexing
    tunnel: "<tr><td colspan=\"2\" style=\"background-color: #DDD;\"><BIG>%s</BIG>(<span class=AccScope>%s</span>)</td></tr>\n<tr><td width=\"50px\">&nbsp;</td><td>%s</td></tr>" -> [w33]
    shift-right: [w31] -> w13
    shift-left: "" -> [w32]
    tunnel: string[] ["Modifiers", "Owner", "Parent", "Generics", "Documentation", "Attributes", "Enum", "Struct", "Methods"] -> [w28]
    tunnel: "MissingClasses" -> [w23]
    tunnel: "InterfacesThatWillUseInheritance" -> [w22]
    tunnel: "InterfacesThatWillUseInheritance" -> [w21]
    tunnel: "<strike>%s</strike>&nbsp;<span class=ModifiedText>%s</span>: %s" ("format string") -> [w16]
    n2 = Unbundle By Name(w27) -> ("ClassName"=w18:string, "ClassType"=w19:T9, "AccessScope"=w24:T2)
    n3 = Search 1D Array(1D array=w21, element=w18) -> (index of element=w20:i32)  [unwired: 1 in]
    n4 = for {
      tunnel: w28 -> [w48] mode=indexing
      tunnel: w27 -> [w47]
      tunnel: [w46] -> w26 mode=indexing
      tunnel: w18 -> [w45]
      tunnel: w23 -> [w44]
      tunnel: w22 -> [w43]
      n5 = case shown="\"Parent\"" w48 {
        selector: w48 -> [_ w53 w69 w83 w122 w164 w183 w237 w345 w354]
        tunnel: w47 -> [_ w52 w68 w82 w121 w163 w182 w236 w344 w353]
        tunnel: [_ w51 w67 w81 w120 w162 w181 w235 w343 w352] -> w46
        tunnel: w45 -> [_ _ _ _ _ _ _ w232 _ _]
        tunnel: w44 -> [_ _ _ _ _ w159 w178 w231 _ _]
        tunnel: w43 -> [_ _ _ w78 _ _ _ _ _ _]
        frame Default {
        }
        frame "Modifiers" {
          n6 = Unbundle By Name(w52) -> ("Modifiers"=w50:T3[])
          n7 = Empty Array?(array=w50) -> (empty?=w49:bool)
          n8 = case shown="False" w49 {
            tunnel: w53 -> [w61 _]
            tunnel: [w56 _] -> w51
            tunnel: w50 -> [w55 _]
            frame False {
              n9 = for {
                tunnel: w55 -> [w64] mode=indexing
                tunnel: [w63] -> w60 mode=indexing
                n10 = Format Into String(w64) -> (resulting string=w63:string)  [unwired: 3 in, 1 out]
              }
              n11 = Array To Spreadsheet String(delimiter (Tab)=",", array=w60, 3:"%s" ("format string")) -> (spreadsheet string=w54:string)
              n12 = call <vilib>:"Trim Whitespace.vi"("string"=w54) -> ("trimmed string"=w57:string)  [unwired: 1 in]
              n13 = Format Into String(format string="<tr><td width=\"50px\">&nbsp;</td><td><b>%s:</b></td><td><span class=AccScope>%s</span></td></tr>", w61, w57) -> (resulting string=w56:string)  [unwired: 2 in, 1 out]
            }
            frame True {
            }
          }
        }
        frame "Generics" {
          n14 = Unbundle By Name(w68) -> ("Generics"=w66:string[])
          n15 = Empty Array?(array=w66) -> (empty?=w65:bool)
          n16 = case shown="False" w65 {
            tunnel: w69 -> [w76 _]
            tunnel: [w71 _] -> w67
            tunnel: w66 -> [w70 _]
            frame False {
              n17 = Array To Spreadsheet String(delimiter (Tab)=",", array=w70, 3:"%s" ("format string")) -> (spreadsheet string=w73:string)
              n18 = call <vilib>:"Trim Whitespace.vi"("string"=w73) -> ("trimmed string"=w72:string)  [unwired: 1 in]
              n19 = Format Into String(format string="<tr><td width=\"50px\">&nbsp;</td><td><b>%s:</b></td><td>%s</td></tr>", w76, w72) -> (resulting string=w71:string)  [unwired: 2 in, 1 out]
            }
            frame True {
            }
          }
        }
        frame "Parent" {
          n20 = Unbundle By Name(w82) -> ("ParentClasses"=w80:T8[])
          n21 = Empty Array?(array=w80) -> (empty?=w79:bool)
          n22 = case shown="False" w79 {
            tunnel: w83 -> [w93 _]
            tunnel: [w87 _] -> w81
            tunnel: w80 -> [w86 _]
            tunnel: w78 -> [w85 _]
            frame False {
              n23 = for {
                tunnel: w86 -> [w104] mode=indexing
                tunnel: [w105] -> w92 mode=indexing
                tunnel: w85 -> [w103]
                tunnel: "<strike>%s</strike>&nbsp;<span class=ModifiedText>%s</span>: %s" ("format string") -> [w95]
                n24 = Unbundle(w104) -> ("ClassName"=w102:string, "ClassType"=w101:T9)
                n25 = Search 1D Array(1D array=w103, element=w102) -> (index of element=w99:i32)  [unwired: 1 in]
                n26 = Equal?(x=w101, y=GDSString_ClassType."Interface") -> (x = y?=w98:bool)
                n27 = Greater Or Equal To 0?(x=w99) -> (x >= 0?=w97:bool)
                n28 = And(x=w98, y=w97) -> (x .and. y?=w96:bool)
                n29 = case shown="True" w96 {
                  tunnel: [w110 w117] -> w105
                  tunnel: w102 -> [w107 w116]
                  tunnel: w101 -> [w106 _]
                  tunnel: w95 -> [_ w113]
                  frame False {
                    n30 = case shown="\"Interface\"" w106 {
                      selector: w106 -> [w111 _]
                      tunnel: [w111 GDSString_ClassType."Class" ("ClassType")] -> w109
                      frame "Interface" {
                      }
                      frame Default {
                      }
                    }
                    n31 = Format Into String(format string="%s : %s", w109, w107) -> (resulting string=w110:string)  [unwired: 2 in, 1 out]
                  }
                  frame True {
                    n32 = Format Into String(format string=w113, GDSString_ClassType."Interface" ("y"), GDSString_ClassType."Class" ("y"), w116) -> (resulting string=w117:string)  [unwired: 2 in, 1 out]
                  }
                }
              }
              n33 = Array To Spreadsheet String(delimiter (Tab)="<br>", array=w92, 3:"%s" ("format string")) -> (spreadsheet string=w89:string)
              n34 = call <vilib>:"Trim Whitespace.vi"("string"=w89) -> ("trimmed string"=w88:string)  [unwired: 1 in]
              n35 = Format Into String(format string="<tr><td width=\"50px\">&nbsp;</td><td><b>%s:</b></td><td>%s</td></tr>", w93, w88) -> (resulting string=w87:string)  [unwired: 2 in, 1 out]
            }
            frame True {
            }
          }
        }
        frame "Enum" {
          n36 = Unbundle By Name(w121) -> ("Enums"=w119:T11[])
          n37 = Empty Array?(array=w119) -> (empty?=w118:bool)
          n38 = case shown="False" w118 {
            tunnel: w122 -> [w130 _]
            tunnel: [w124 _] -> w120
            tunnel: w119 -> [w123 _]
            frame False {
              n39 = for {
                tunnel: w123 -> [w148] mode=indexing
                tunnel: [w149] -> w129 mode=indexing
                n40 = Unbundle(w148) -> ("Name"=w147:string, "AccessScope"=w145:T2, "Modifiers"=w144:T3[], "Items"=w135:string[], "Documentation"=w133:string)
                n41 = for {
                  tunnel: w144 -> [w158] mode=indexing
                  tunnel: [w157] -> w143 mode=indexing
                  n42 = Format Into String(format string="%s,", w158) -> (resulting string=w157:string)  [unwired: 2 in, 1 out]
                }
                n43 = Concatenate Strings(w143) -> (w142:string)
                n44 = Array To Spreadsheet String(delimiter (Tab)=",", array=w135, 3:"%s" ("format string")) -> (spreadsheet string=w136:string)
                n45 = case shown="\"False\", Default" w133 {
                  selector: w133 -> [w152 _]
                  tunnel: [w151 _] -> w132
                  frame "False", Default {
                    n46 = Format Into String(format string="<br><b>Documentation:</b>&nbsp;<div class=doc>%s</div>", w152) -> (resulting string=w151:string)  [unwired: 2 in, 1 out]
                  }
                  frame "" {
                  }
                }
                n47 = Match Pattern(string=w142, regular expression=",$") -> (before substring=w140:string)  [unwired: 1 in, 3 out]
                n48 = call <vilib>:"Trim Whitespace.vi"("string"=w136) -> ("trimmed string"=w134:string)  [unwired: 1 in]
                n49 = case shown="Default" w140 {
                  selector: w140 -> [w155 _]
                  tunnel: [w153 _] -> w139
                  frame Default {
                    n50 = Format Into String(format string="(%s)", w155) -> (resulting string=w153:string)  [unwired: 2 in, 1 out]
                  }
                  frame "" {
                  }
                }
                n51 = Format Into String(format string="<span class=AccScope>%s</span> : %s<span class=AccScope>%s</span> : %s%s", w145, w147, w139, w134, w132) -> (resulting string=w149:string)  [unwired: 2 in, 1 out]
              }
              n52 = Array To Spreadsheet String(delimiter (Tab)="<br>", array=w129, 3:"%s" ("format string")) -> (spreadsheet string=w126:string)
              n53 = call <vilib>:"Trim Whitespace.vi"("string"=w126) -> ("trimmed string"=w125:string)  [unwired: 1 in]
              n54 = Format Into String(format string="<tr><td width=\"50px\">&nbsp;</td><td><b>%s:</b></td><td>%s</td></tr>", w130, w125) -> (resulting string=w124:string)  [unwired: 2 in, 1 out]
            }
            frame True {
            }
          }
        }
        frame "Attributes" {
          n55 = Unbundle By Name(w163) -> ("Attributes"=w161:T5[])
          n56 = Empty Array?(array=w161) -> (empty?=w160:bool)
          n57 = case shown="False" w160 {
            tunnel: w164 -> [w173 _]
            tunnel: [w167 _] -> w162
            tunnel: w161 -> [w166 _]
            tunnel: w159 -> [w165 _]
            frame False {
              n58 = for {
                tunnel: w166 -> [w176] mode=indexing
                tunnel: [w177] -> w172 mode=indexing
                tunnel: w165 -> [w175]
                n59 = call <resource>:"ConvertTextBasedCodeToLabVIEW_AttToHtml.vi"("MissingClasses"=w175, "DataType"=w176) -> ("String"=w177:string)  [unwired: 9 in]
              }
              n60 = Array To Spreadsheet String(delimiter (Tab)="<br>", array=w172, 3:"%s" ("format string")) -> (spreadsheet string=w169:string)
              n61 = call <vilib>:"Trim Whitespace.vi"("string"=w169) -> ("trimmed string"=w168:string)  [unwired: 1 in]
              n62 = Format Into String(format string="<tr><td width=\"50px\">&nbsp;</td><td><b>%s:</b></td><td>%s</td></tr>", w173, w168) -> (resulting string=w167:string)  [unwired: 2 in, 1 out]
            }
            frame True {
            }
          }
        }
        frame "Struct" {
          n63 = Unbundle By Name(w182) -> ("Structs"=w179:T12[])
          n64 = Empty Array?(array=w179) -> (empty?=w180:bool)
          n65 = case shown="False" w180 {
            tunnel: w183 -> [w192 _]
            tunnel: [w186 _] -> w181
            tunnel: w179 -> [w185 _]
            tunnel: w178 -> [w184 _]
            frame False {
              n66 = for {
                tunnel: [w208] -> w191 mode=indexing
                tunnel: w185 -> [w206] mode=indexing
                tunnel: w184 -> [w194]
                n67 = Unbundle By Name(w206) -> ("Name"=w199:string, "AccessScope"=w205:T2, "Modifiers"=w200:T3[], "Documentation"=w197:string)
                n68 = Unbundle By Name(w206) -> ("Items"=w209:T5[])
                n69 = for {
                  tunnel: w209 -> [w222] mode=indexing
                  tunnel: [w221] -> w210 mode=indexing
                  tunnel: w194 -> [w220]
                  n70 = Unbundle(w222) -> ("Name"=w224:string, "DataType"=w227:T6, "ArrayDim"=w228:i32, "AccessScope"=w223:T2)  [unwired: 3 out]
                  n71 = for {
                    N: w228 -> [_]
                    tunnel: ["[]"] -> w226 mode=indexing
                  }
                  n72 = Concatenate Strings(w226) -> (w225:string)
                  n73 = call <resource>:"ConvertTextBasedCodeToLabVIEW_AttToHtml.vi"("MissingClasses"=w220, "DataType"=w222) -> ("String"=w221:string)  [unwired: 9 in]
                  n74 = Format Into String(format string="<span class=AccScope>%s</span> %s%s : %s", w223, w227, w225, w224) -> ()  [unwired: 2 in, 2 out]
                }
                n75 = for {
                  tunnel: w200 -> [w219] mode=indexing
                  tunnel: [w218] -> w204 mode=indexing
                  n76 = Format Into String(format string="%s,", w219) -> (resulting string=w218:string)  [unwired: 2 in, 1 out]
                }
                n77 = case shown="\"False\", Default" w197 {
                  selector: w197 -> [w213 _]
                  tunnel: [w212 _] -> w196
                  frame "False", Default {
                    n78 = Format Into String(format string="<br><b>Documentation:</b>&nbsp;<div class=doc>%s</div>", w213) -> (resulting string=w212:string)  [unwired: 2 in, 1 out]
                  }
                  frame "" {
                  }
                }
                n79 = Concatenate Strings(w204) -> (w203:string)
                n80 = Match Pattern(string=w203, regular expression=",$") -> (before substring=w201:string)  [unwired: 1 in, 3 out]
                n81 = case shown="Default" w201 {
                  selector: w201 -> [w216 _]
                  tunnel: [w214 _] -> w198
                  frame Default {
                    n82 = Format Into String(format string="(%s)", w216) -> (resulting string=w214:string)  [unwired: 2 in, 1 out]
                  }
                  frame "" {
                  }
                }
                n83 = Format Into String(format string="<span class=AccScope>%s</span> %s<span class=AccScope>%s</span>%s", w205, w199, w198, w196) -> (resulting string=w195:string)  [unwired: 2 in, 1 out]
                n84 = Build Array (concatenate)(w195, w210) -> (w208:string[])
              }
              n85 = Array To Spreadsheet String(delimiter (Tab)="<br>", array=w191, 3:"%s" ("format string")) -> (spreadsheet string=w188:string)
              n86 = call <vilib>:"Trim Whitespace.vi"("string"=w188) -> ("trimmed string"=w187:string)  [unwired: 1 in]
              n87 = Format Into String(format string="<tr><td width=\"50px\">&nbsp;</td><td><b>%s:</b></td><td>%s</td></tr>", w192, w187) -> (resulting string=w186:string)  [unwired: 2 in, 1 out]
            }
            frame True {
            }
          }
        }
        frame "Methods" {
          n88 = Unbundle By Name(w236) -> ("Methods"=w233:T4[])
          n89 = Empty Array?(array=w233) -> (empty?=w234:bool)
          n90 = case shown="False" w234 {
            tunnel: w237 -> [w247 _]
            tunnel: [w241 _] -> w235
            tunnel: w233 -> [w240 _]
            tunnel: w232 -> [w239 _]
            tunnel: w231 -> [w238 _]
            frame False {
              n91 = for {
                tunnel: [w277] -> w246 mode=indexing
                tunnel: w240 -> [w286] mode=indexing
                tunnel: w239 -> [w254]
                tunnel: w238 -> [w249]
                w271 = "void" ("y")
                n92 = Unbundle By Name(w286) -> ("MethodName"=w255:string, "GetProperty"=w263:T7, "SetProperty"=w262:T7, "AccessScope"=w264:T2, "MethodArguments"=w265:T5[], "Modifiers"=w281:T3[], "MethodDocumentation"=w278:string, "ReturnType"=w276:T5)
                n93 = Unbundle By Name(w276) -> ("DataTypeString"=w273:string, "Name"=w272:string, "DataType"=w267:T6, "ArrayDim"=w274:i32)
                n94 = Equal?(x=w254, y=w255) -> (x = y?=w253:bool)
                n95 = Unbundle(w263) -> ("Active"=w258:bool, "AccessScope"=w260:T2)  [unwired: 1 out]
                n96 = Unbundle(w262) -> ("Active"=w257:bool, "AccessScope"=w259:T2)  [unwired: 1 out]
                n97 = case shown="\"False\", Default" w278 {
                  selector: w278 -> [w334 _]
                  tunnel: [w333 _] -> w279
                  frame "False", Default {
                    n98 = Format Into String(format string="<br><b>Documentation:</b>&nbsp;<div class=doc>%s</div>", w334) -> (resulting string=w333:string)  [unwired: 2 in, 1 out]
                  }
                  frame "" {
                  }
                }
                n99 = for {
                  N: w274 -> [_]
                  tunnel: ["[]"] -> w275 mode=indexing
                }
                n100 = Or(x=w258, y=w257) -> (x .or. y?=w261:bool)
                n101 = Equal?(x=w273, y=w271) -> (x = y?=w270:bool)
                n102 = for {
                  tunnel: w281 -> [w340] mode=indexing
                  tunnel: [w339] -> w285 mode=indexing
                  n103 = Format Into String(format string="%s,", w340) -> (resulting string=w339:string)  [unwired: 2 in, 1 out]
                }
                n104 = Equal?(x=w272, y=w271) -> (x = y?=w269:bool)
                n105 = case shown="False" w261 {
                  tunnel: w265 -> [w295 _]
                  tunnel: w260 -> [_ w321]
                  tunnel: w259 -> [_ w317]
                  tunnel: w258 -> [_ w315]
                  tunnel: w257 -> [_ w313]
                  tunnel: [w289 w300] -> w256
                  tunnel: w249 -> [w288 _]
                  frame False {
                    n106 = for {
                      tunnel: w295 -> [w299] mode=indexing
                      tunnel: [w298] -> w294 mode=indexing
                      tunnel: w288 -> [w296]
                      n107 = call <resource>:"ConvertTextBasedCodeToLabVIEW_AttToHtml.vi"("MissingClasses"=w296, "ShowAccesScope(True)"=FALSE, "DataType"=w299) -> ("String"=w298:string)  [unwired: 8 in]
                    }
                    n108 = Array To Spreadsheet String(delimiter (Tab)=",", array=w294, 3:"%s" ("format string")) -> (spreadsheet string=w290:string)
                    n109 = Format Into String(format string="(%s)", w290) -> (resulting string=w289:string)  [unwired: 2 in, 1 out]
                  }
                  frame True {
                    w309 = string[] [] ("f")
                    n110 = case shown="\"public\"" w321 {
                      selector: w321 -> [_ w325]
                      tunnel: [_ w324] -> w318
                      frame "public" {
                      }
                      frame Default {
                        n111 = Format Into String(w325) -> (resulting string=w324:string)  [unwired: 3 in, 1 out]
                      }
                    }
                    n112 = case shown="\"public\"" w317 {
                      selector: w317 -> [_ w323]
                      tunnel: [_ w322] -> w316
                      frame "public" {
                      }
                      frame Default {
                        n113 = Format Into String(w323) -> (resulting string=w322:string)  [unwired: 3 in, 1 out]
                      }
                    }
                    n114 = Format Into String(format string="%sget", w318) -> (resulting string=w314:string)  [unwired: 2 in, 1 out]
                    n115 = Format Into String(format string="%sset", w316) -> (resulting string=w312:string)  [unwired: 2 in, 1 out]
                    n116 = Build Array(w314) -> (w311:string[])
                    n117 = Build Array(w312) -> (w310:string[])
                    n118 = Select(t=w311, s=w315, f=w309) -> (s? t:f=w308:string[])
                    n119 = Select(t=w310, s=w313, f=w309) -> (s? t:f=w307:string[])
                    n120 = Build Array (concatenate)(w308, w307) -> (w306:string[])
                    n121 = Array To Spreadsheet String(delimiter (Tab)=", ", array=w306, 3:"%s" ("format string")) -> (spreadsheet string=w303:string)
                    n122 = call <vilib>:"Trim Whitespace.vi"("string"=w303) -> ("trimmed string"=w301:string)  [unwired: 1 in]
                    n123 = Format Into String(format string="{%s}", w301) -> (resulting string=w300:string)  [unwired: 2 in, 1 out]
                  }
                }
                n124 = Concatenate Strings(w275) -> (w266:string)
                n125 = Or(x=w270, y=w269) -> (x .or. y?=w268:bool)
                n126 = Concatenate Strings(w285) -> (w284:string)
                n127 = Match Pattern(string=w284, regular expression=",$") -> (before substring=w282:string)  [unwired: 1 in, 3 out]
                n128 = case shown="True" w268 {
                  tunnel: w267 -> [w327 _]
                  tunnel: w266 -> [w328 _]
                  tunnel: [w326 "void" ("y")] -> w251
                  frame False {
                    n129 = Format Into String(format string="%s%s", w327, w328) -> (resulting string=w326:string)  [unwired: 2 in, 1 out]
                  }
                  frame True {
                  }
                }
                n130 = case shown="Default" w282 {
                  selector: w282 -> [w337 _]
                  tunnel: [w335 _] -> w280
                  frame Default {
                    n131 = Format Into String(format string="(%s)", w337) -> (resulting string=w335:string)  [unwired: 2 in, 1 out]
                  }
                  frame "" {
                  }
                }
                n132 = Select(t="", s=w253, f=w251) -> (s? t:f=w252:string)
                n133 = Format Into String(format string="<span class=AccScope>%s%s</span> %s <b>%s</b> %s%s", w264, w280, w252, w255, w256, w279) -> (resulting string=w277:string)  [unwired: 2 in, 1 out]
              }
              n134 = Array To Spreadsheet String(delimiter (Tab)="<br>", array=w246, 3:"%s" ("format string")) -> (spreadsheet string=w243:string)
              n135 = call <vilib>:"Trim Whitespace.vi"("string"=w243) -> ("trimmed string"=w242:string)  [unwired: 1 in]
              n136 = Format Into String(format string="<tr><td width=\"50px\">&nbsp;</td><td><b>%s:</b></td><td>%s</td></tr>", w247, w242) -> (resulting string=w241:string)  [unwired: 2 in, 1 out]
            }
            frame True {
            }
          }
        }
        frame "Owner" {
          n137 = Unbundle By Name(w344) -> ("Owner"=w341:string, "OwnerType"=w342:T10)
          n138 = case shown="\"Class\", \"Package/NameSpace\"" w342 {
            tunnel: w345 -> [_ w348]
            tunnel: [_ w347] -> w343
            tunnel: w342 -> [_ _]
            tunnel: w341 -> [_ w346]
            frame "NoOwner", Default {
            }
            frame "Class", "Package/NameSpace" {
              n139 = Format Into String(format string="<tr><td width=\"50px\">&nbsp;</td><td><b>%s:</b></td><td>%s</td></tr>", w348, w346) -> (resulting string=w347:string)  [unwired: 2 in, 1 out]
            }
          }
        }
        frame "Documentation" {
          n140 = Unbundle By Name(w353) -> ("ClassDocumentation"=w351:string)
          n141 = Empty String/Path?(string/path=w351) -> (empty?=w350:bool)
          n142 = case shown="False" w350 {
            tunnel: w354 -> [_ w357]
            tunnel: [_ w356] -> w352
            tunnel: w351 -> [_ w355]
            frame True {
            }
            frame False {
              n143 = Format Into String(format string="<tr><td width=\"50px\">&nbsp;</td><td><b>%s:</b></td><td><div class=doc>%s</div></td></tr>", w357, w355) -> (resulting string=w356:string)  [unwired: 2 in, 1 out]
            }
          }
        }
      }
    }
    n144 = case shown="Default" w20 {
      tunnel: w19 -> [w36 _]
      tunnel: w18 -> [w35 w42]
      tunnel: [w34 w41] -> w17
      tunnel: w16 -> [_ w40]
      frame -1 {
        n145 = Format Into String(format string="%s : %s", w36, w35) -> (resulting string=w34:string)  [unwired: 2 in, 1 out]
      }
      frame Default {
        n146 = Format Into String(format string=w40, GDSString_ClassType."Interface" ("y"), GDSString_ClassType."Class" ("y"), w42) -> (resulting string=w41:string)  [unwired: 2 in, 1 out]
      }
    }
    n147 = Concatenate Strings(w26) -> (w25:string)
    n148 = Format Into String(format string="<table class=SubTable>\n%s\n</table>", w25) -> (resulting string=w29:string)  [unwired: 2 in, 1 out]
    n149 = Format Into String(format string=w33, initial string=w32, w17, w24, w29) -> (resulting string=w31:string)  [unwired: 1 in, 1 out]
  }
  n150 = Format Into String(format string="<table class=MainTable>\n%s\n</table>", w13) -> (resulting string=w10:string)  [unwired: 2 in, 1 out]
  n151 = Format Into String(format string="<!DOCTYPE html>\n<html>\n    \n    <head>\n        <meta charset=\"utf-8\">\n        <title>CLASS OVERVIEW</title>\n    </head>\n    <style>\n    \n    html {\n    background-color: #e6e9e9;\n    background-image: -webkit-linear-gradient(270deg,rgb(230,233,233) 0%%,rgb(216,221,221) 100%%);\n    background-image: linear-gradient(270deg,rgb(230,233,233) 0%%,rgb(216,221,221) 100%%);\n    -webkit-font-smoothing: antialiased;\n}\n\nbody {\n    margin: 0 auto;\n    padding: 2em 2em 4em;\n    max-width: 800px;\n    font-family: \"Helvetica Neue\", Helvetica, Arial, sans-serif;\n    font-size: 16px;\n    line-height: 1.5em;\n    color: #545454;\n    background-color: #ffffff;\n    box-shadow: 0 0 2px rgba(0, 0, 0, 0.06);\n}\n\nh1, h2, h3, h4, h5, h6 {\n    color: #222;\n    font-weight: 600;\n    line-height: 1.3em;\n}\n\nh2 {\n    margin-top: 1.3em;\n}\n\na {\n    color: #0083e8;\n}\n\ntr {\n    vertical-align: top;\n}        \n\n.doc {\n    color: #208820;\nfont-style: italic;\n}\n\n.LVClassName {\n    color: #208820;\nfont-style: italic;\n}\n\n.MissingLVClassName\n{\n    color: #FF2020;\nfont-style: italic;\n}\n\n.AccScope {\n    color: #2020FF;\n}\n\n.ModifiedText {\n    color: #FF0000;\n}\n\ntable, th, td {\n    border: 0px;\n    border-collapse: collapse;\n}\n\n-.SubTable tr:nth-child(even) {background-color: #CCC}\n-.SubTable tr:nth-child(odd) {background-color: #FFF}     \n\n-.MainTable tr:nth-child(even) {background-color: #FFF}\n-.MainTable tr:nth-child(odd) {background-color: #DDD}     \n        \n    </style>\n    <body>\n        \n        <h1>CLASS OVERVIEW</h1>\n  %s      \n     \n        \n    </body>\n</html>\n", w10) -> (resulting string=w8:string)  [unwired: 2 in, 1 out]
  n152 = Write to Text File(file (use dialog)="appended path in", text=w8, error in="error in (no error)") -> (error out=w5:errorcluster)  [unwired: 1 in, 2 out]
  "error out" <- w5
  n153 = disable-structure shown="Enabled" {
    disable-tunnel: "appended path in" -> [_ w360]
    disable-tunnel: w5 -> [_ w359]
    frame Enabled {
    }
    frame Disabled {
      n154 = call-poly <vilib>:"Open URL in Default Browser.vi"("error in (no error)"=w359, "path"=w360) -> ()  [unwired: 4 in, 2 out]
    }
  }
  "appended path out" <- "appended path in"
